vi "QCP_GetDbl.vi"(8 "error in (no error)":errorcluster, 10 "Value Name":string, 11 "QCP_DevRef_In":T1) -> (0 "error out":errorcluster, 2 "Value":dbl, 3 "QCP_DevRef_Out":T1)   [LabVIEW 2016]
uses:
  <userlib>/836-libraries/System/QCP_V2/QCPSupportCode/QCP_RefNum.ctl
  <userlib>/836-libraries/System/QCP_V2/QCPSupportCode/QCPData.ctl
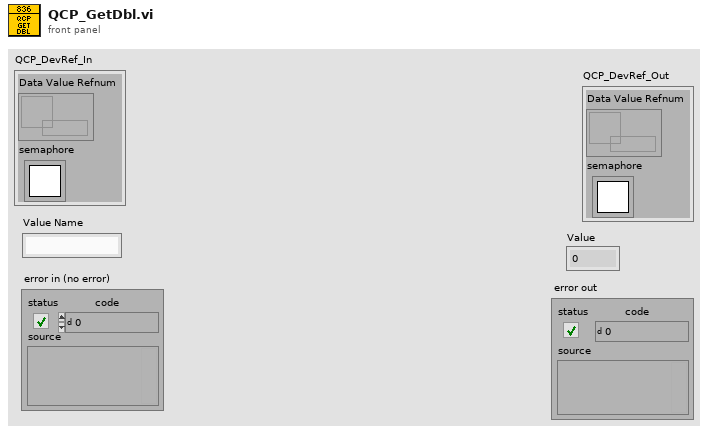
[diagram p1: front panel]
types:
  T1 = typedef "QCP_RefNum.ctl" = cluster{"Data Value Refnum":refnum<data-value>, "semaphore":T2}
  T2 = typedef "Semaphore RefNum" = refnum<k1>
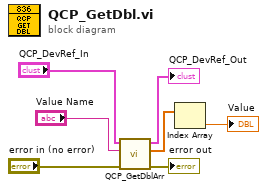
[diagram p0: block diagram]
diagram:
  n1 = call <userlib>:"QCP_GetDblArr.vi"("error in (no error)"="error in (no error)", "Value Name"="Value Name", "QCP_DevRef_In"="QCP_DevRef_In") -> ("error out"=→"error out":errorcluster, "Values"=w2:dbl[], "QCP_DevRef_Out"=→"QCP_DevRef_Out":T1)  [unwired: 6 in]
  n2 = Index Array(array=w2) -> (element=→"Value":dbl)  [unwired: 1 in]
